vi "Culab Complex Process.vi"(11 "X size":i32=16384) -> (3 "Culab Time":dbl=1.016902899999991)   [LabVIEW 2020]
uses:
  <vilib>/Ngene/CuLab - GPU Accelerated Toolkit/Toolkit/Low_Level/Tensor_Classes/T_Children/T1D/T1D_Children/T1D_CSG/Create_Push.vi
  <vilib>/Ngene/CuLab - GPU Accelerated Toolkit/Toolkit/Low_Level/Tensor_Classes/T_Children/T0D/T0D_Children/T0D_CSG/Create.vi
  <vilib>/Ngene/CuLab - GPU Accelerated Toolkit/Toolkit/Low_Level/Tensor_Classes/T_Children/T0D/T0D_Children/T0D_CSG/Pull.vi
  <vilib>/Ngene/CuLab - GPU Accelerated Toolkit/Toolkit/CuLab.lvlib
  <vilib>/Ngene/CuLab - GPU Accelerated Toolkit/Toolkit/Low_Level/Tensor_Classes/T_Children/T1D/T1D_Children/T1D_CSG/T1D_CSG.lvclass
  <vilib>/Ngene/CuLab - GPU Accelerated Toolkit/Toolkit/Low_Level/Tensor_Classes/T_Children/T0D/T0D_Children/T0D_CSG/T0D_CSG.lvclass
  <vilib>/Analysis/NI_AALBase.lvlib
panel:
  out "Dest out":csg=7.867303e+19-1.7997234e+21i
  in  "nb_loop":i32=6
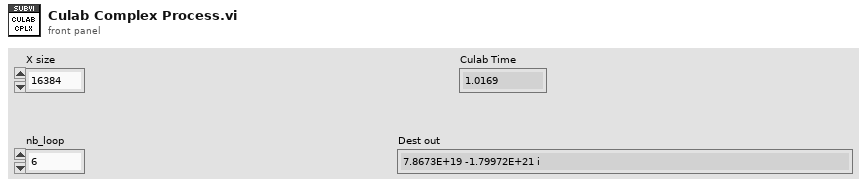
[diagram p1: front panel]
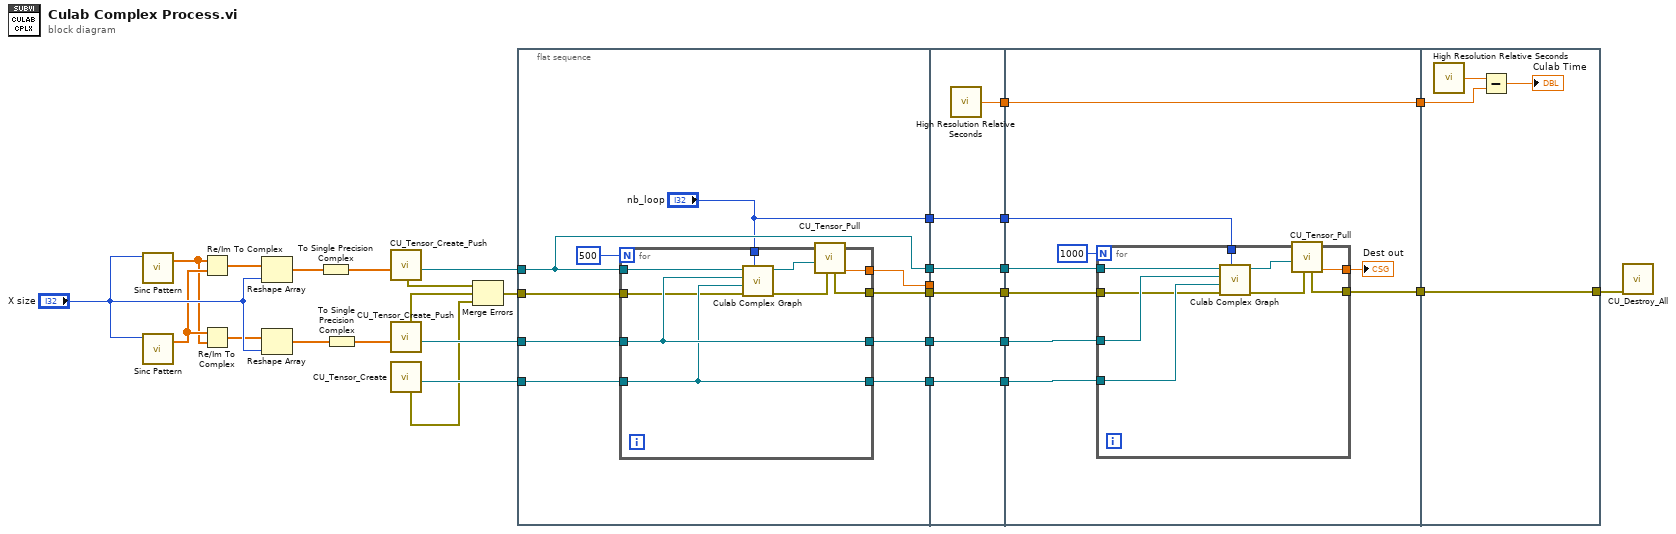
[diagram p0: block diagram]
diagram:
  n1 = call <vilib>:"Sinc Pattern.vi"("samples"="X size") -> ("Sinc Pattern"=w10:dbl[])  [unwired: 3 in, 1 out]
  n2 = call <vilib>:"Sinc Pattern.vi"("samples"="X size") -> ("Sinc Pattern"=w11:dbl[])  [unwired: 3 in, 1 out]
  n3 = Re/Im To Complex(1:w11, 2:w10) -> (0:w12:cdb[])
  n4 = Re/Im To Complex(1:w10, 2:w11) -> (0:w9:cdb[])
  n5 = Reshape Array(w12, "X size") -> (w8:cdb[])
  n6 = Reshape Array(w9, "X size") -> (w7:cdb[])
  n7 = To Single Precision Complex(1:w8) -> (0:w6:csg[])
  n8 = To Single Precision Complex(1:w7) -> (0:w5:csg[])
  n9 = call-poly <vilib>:"CU_Tensor_Create_Push.vi"("CPU_Data_1D_CSG"=w6) -> ("T1D_CSG out"=w28:refnum<class "T1D_CSG.lvclass">, "error out"=w2:errorcluster)  [unwired: 9 in]
  n10 = call-poly <vilib>:"CU_Tensor_Create_Push.vi"("CPU_Data_1D_CSG"=w5) -> ("T1D_CSG out"=w27:refnum<class "T1D_CSG.lvclass">, "error out"=w3:errorcluster)  [unwired: 9 in]
  n11 = call-poly <vilib>:"CU_Tensor_Create.vi"() -> ("T0D_CSG out"=w26:refnum<class "T0D_CSG.lvclass">, "error out"=w4:errorcluster)  [unwired: 10 in]
  n12 = Merge Errors(w2, w3, w4) -> (w1:errorcluster)
  n13 = flat-sequence {
    tunnel: w26 -> [w36]
    tunnel: w27 -> [w41]
    tunnel: w28 -> [w39]
    tunnel: [w40] -> w25
    tunnel: [w39] -> w24
    tunnel: [w37] -> w22
    tunnel: [w35] -> w20
    tunnel: [w34] -> w18
    tunnel: ["nb_loop"] -> w14
    tunnel: w1 -> [w32]
    tunnel: [w56] -> w31
    tunnel: [w55] -> w30
    tunnel: w25 -> [_]
    tunnel: w24 -> [w55]
    tunnel: [w54] -> w23
    tunnel: w22 -> [w54]
    tunnel: [w53] -> w21
    tunnel: w20 -> [w53]
    tunnel: [w52] -> w19
    tunnel: w18 -> [w52]
    tunnel: [w51] -> w15
    tunnel: w14 -> [w51]
    tunnel: w31 -> [w65]
    tunnel: [w65] -> w29
    tunnel: w30 -> [w62]
    tunnel: w23 -> [w58]
    tunnel: w21 -> [w64]
    tunnel: w19 -> [w63]
    tunnel: [w60] -> w16
    tunnel: w15 -> [w59]
    tunnel: w29 -> [w77]
    tunnel: [w75] -> w17
    tunnel: w16 -> [w75]
    frame #0 {
      n14 = for {
        N: 500 -> [_]
        tunnel: w41 -> [w46]
        tunnel: [w50] -> w40
        tunnel: w39 -> [w48]
        tunnel: [w49] -> w37
        tunnel: w36 -> [w45]
        tunnel: [w46] -> w35
        tunnel: [w45] -> w34
        tunnel: "nb_loop" -> [w44]
        tunnel: w32 -> [w42]
        n15 = call "Culab Complex Graph.vi"("nb_loop"=w44, "error in (no error)"=w42, "C"=w45, "B"=w46, "A"=w48) -> ("error out"=w43:errorcluster, "Dest out"=w47:refnum<class "T0D_CSG.lvclass">)  [unwired: 5 in]
        n16 = call-poly <vilib>:"CU_Tensor_Pull.vi"("error in (no error)"=w43, "T0D_CSG in"=w47) -> ("Dest out"=w50:csg, "error out"=w49:errorcluster)  [unwired: 7 in, 1 out]
      }
    }
    frame #1 {
      n17 = call <vilib>:"High Resolution Relative Seconds.vi"() -> ("relative seconds"=w56:dbl)
    }
    frame #2 {
      n18 = for {
        N: 1000 -> [_]
        tunnel: w64 -> [w71]
        tunnel: [w74] -> w57
        tunnel: w62 -> [w72]
        tunnel: [w73] -> w60
        tunnel: w63 -> [w69]
        tunnel: w59 -> [w68]
        tunnel: w58 -> [w67]
        n19 = call "Culab Complex Graph.vi"("nb_loop"=w68, "error in (no error)"=w67, "C"=w69, "B"=w71, "A"=w72) -> ("error out"=w66:errorcluster, "Dest out"=w70:refnum<class "T0D_CSG.lvclass">)  [unwired: 5 in]
        n20 = call-poly <vilib>:"CU_Tensor_Pull.vi"("error in (no error)"=w66, "T0D_CSG in"=w70) -> ("Dest out"=w74:csg, "error out"=w73:errorcluster)  [unwired: 7 in, 1 out]
      }
      "Dest out" <- w57
    }
    frame #3 {
      n21 = call <vilib>:"High Resolution Relative Seconds.vi"() -> ("relative seconds"=w78:dbl)
      n22 = Subtract(x=w78, y=w77) -> (x-y=→"Culab Time":dbl)
    }
  }
  n23 = call <vilib>:"CU_Destroy_All.vi"("error in"=w17) -> ()  [unwired: 10 in, 1 out]
